vi "Read.vi"(11 "ChannelValue in":refnum<class "StringChannelValue.lvclass">) -> (2 "Channel":refnum<class "StringChannel.lvclass">)   [LabVIEW 2020, in "Vecto.lvlib" / "StringChannelValue.lvclass"]
uses:
  StringChannelValue.lvclass
  StringChannelValue.lvclass/StringChannelValue.ctl
  StringChannel/StringChannel.lvclass
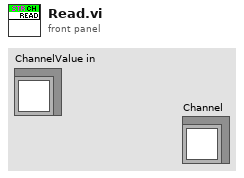
[diagram p1: front panel]
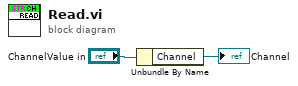
[diagram p0: block diagram]
diagram:
  n1 = Unbundle By Name("ChannelValue in") -> ("Channel"=→"Channel":refnum<class "StringChannel.lvclass">)
